vi "Color Sensor V3 Match Color.vi"(11 "Measured Color":cluster{"R":dbl, "G":dbl, "B":dbl}) -> (1 "Confidence":dbl, 2 "Matched Color":cluster{"R":dbl, "G":dbl, "B":dbl}, 3 "Matched Color Name":string)   [LabVIEW 2019]
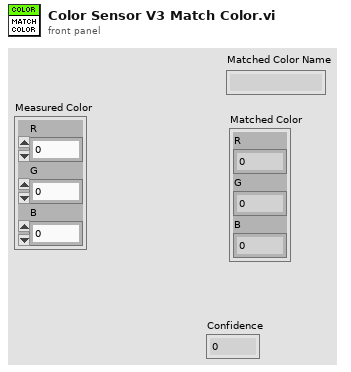
[diagram p1: front panel]
types:
  T1 = typedef "Color Sensor V3 Color Match.ctl" = cluster{"Name":string, "Normalized Color":cluster{"R":dbl, "G":dbl, "B":dbl}}
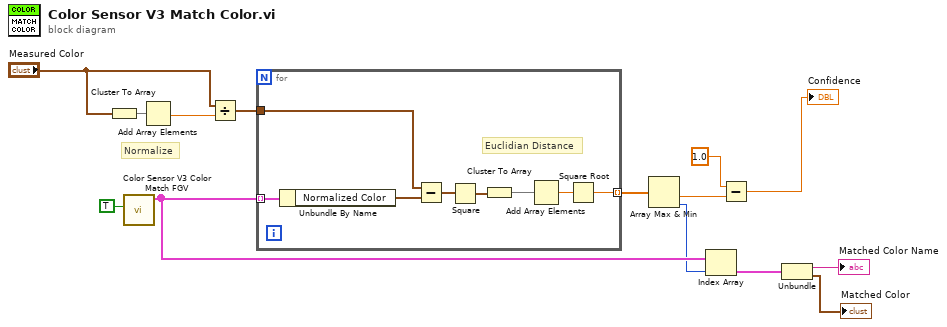
[diagram p0: block diagram]
diagram:
  # "Normalize"
  n1 = Cluster To Array(cluster="Measured Color") -> (array=w4:dbl[])
  n2 = call "Color Sensor V3 Color Match FGV.vi"("Get Only? (F)"=TRUE) -> ("All Match Colors"=w9:T1[])  [unwired: 10 in]
  n3 = Add Array Elements(numeric array=w4) -> (sum=w3:dbl)
  n4 = Divide(x="Measured Color", y=w3) -> (x/y=w1:cluster{"R":dbl, "G":dbl, "B":dbl})
  n5 = for {
    tunnel: w9 -> [w22] mode=indexing
    tunnel: w1 -> [w21]
    tunnel: [w15] -> w13 mode=indexing
    # "Euclidian Distance"
    n6 = Unbundle By Name(w22) -> ("Normalized Color"=w20:cluster{"R":dbl, "G":dbl, "B":dbl})
    n7 = Subtract(x=w21, y=w20) -> (x-y=w19:cluster{"R":dbl, "G":dbl, "B":dbl})
    n8 = Square(x=w19) -> (x^2=w18:cluster{"R":dbl, "G":dbl, "B":dbl})
    n9 = Cluster To Array(cluster=w18) -> (array=w17:dbl[])
    n10 = Add Array Elements(numeric array=w17) -> (sum=w16:dbl)
    n11 = Square Root(x=w16) -> (sqrt(x)=w15:dbl)
  }
  n12 = Array Max & Min(array=w13) -> (min value=w12:dbl, min index (indices)=w8:i32)  [unwired: 2 out]
  n13 = Index Array(array=w9, index=w8) -> (element=w7:T1)
  n14 = Subtract(x=1.0 ("max value"), y=w12) -> (x-y=→"Confidence":dbl)
  n15 = Unbundle(w7) -> ("Name"=→"Matched Color Name":string, "Normalized Color"=→"Matched Color":cluster{"R":dbl, "G":dbl, "B":dbl})
